vi "Read CSV into Table.vi"() -> ()   [LabVIEW 2018]
uses:
  <vilib>/Utility/file.llb/Read From Spreadsheet File (string).vi
panel:
  in  "Path":path=path "C:/ALS Release Tester/Data_Files/2010-9-8_144219 Data Log.txt"
  out "Table Control":string[][](table)
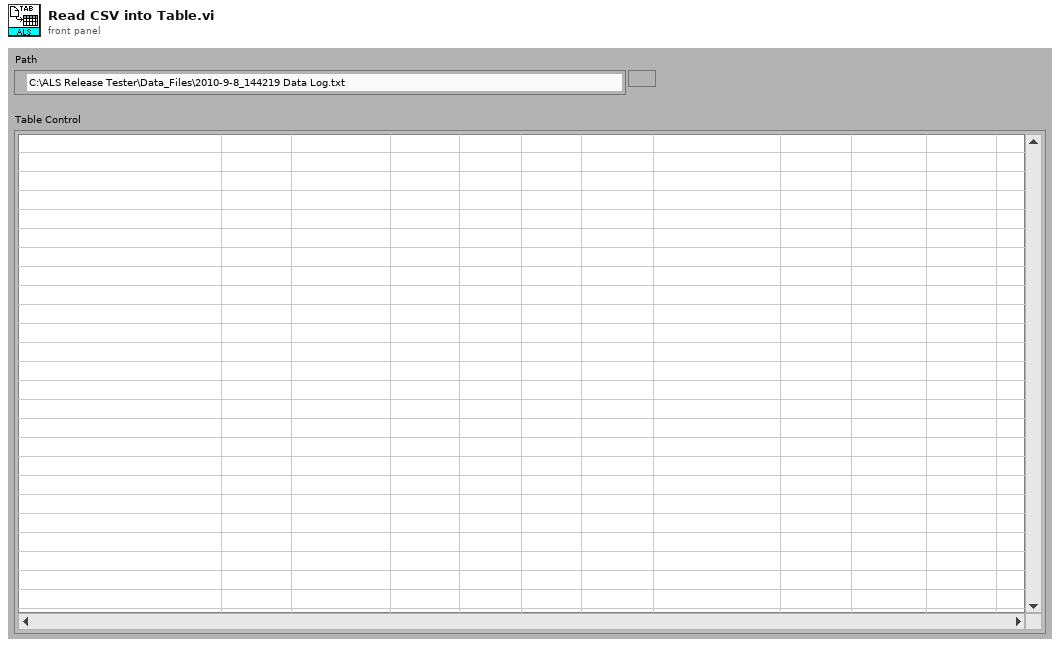
[diagram p1: front panel]
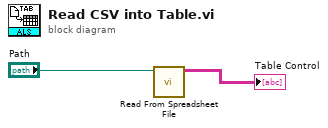
[diagram p0: block diagram]
diagram:
  n1 = call-poly <vilib>:"Read From Spreadsheet File.vi"("file path (dialog if empty)"="Path") -> ("all rows"=→"Table Control":string[][])  [unwired: 6 in, 4 out]
